vi "get_RL.vi"(8 "error in":errorcluster, 9 "Simulation mode":bool, 10 "Average":i32, 11 "Integration Time (ms)":i32) -> (0 "error out":errorcluster, 2 "RL Spectrum":dbl[](array[numeric]), 3 "WL Values":dbl[](array[numeric]))   [LabVIEW 2021]
doc: "Random Laser Project v2.0\nAndré Romero - 2024\nandretec@ifsc.usp.br"
uses:
  Global_v20.vi
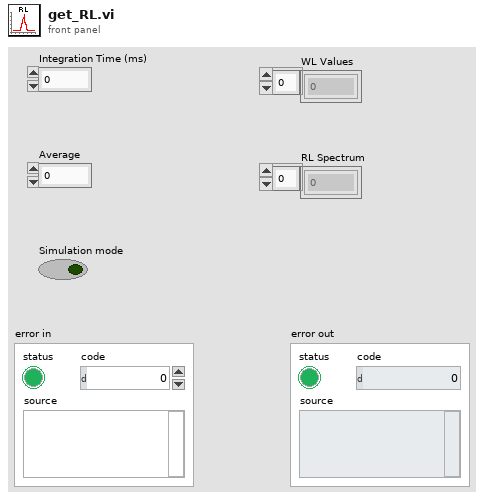
[diagram p1: front panel]
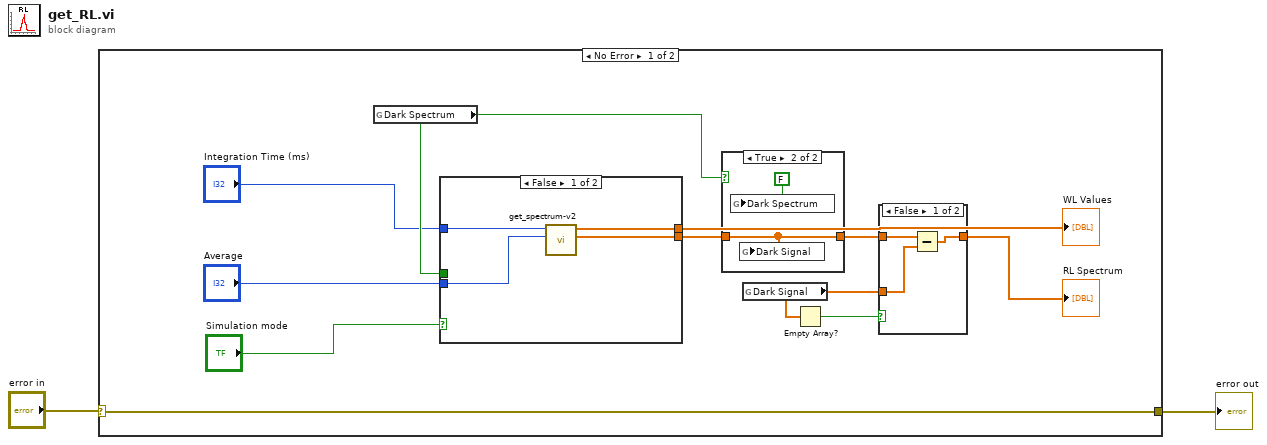
[diagram p0: block diagram]
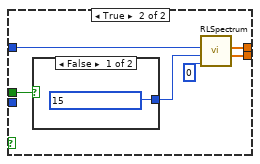
[diagram p3: hidden frame]
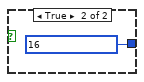
[diagram p4: hidden frame]
diagram:
  n1 = case shown="No Error" "error in" {
    selector: "error in" -> [w3 w33]
    tunnel: [w3 w33] -> w1
    frame No Error {
      n2 = global read "Global_v20.vi" "Dark Spectrum"() -> (w7:bool)
      n3 = case shown="False" "Simulation mode" {
        tunnel: "Integration Time (ms)" -> [w19 w27]
        tunnel: [w21 w26] -> w5
        tunnel: [w20 w25] -> w6
        tunnel: w7 -> [_ w24]
        tunnel: "Average" -> [w18 _]
        frame False {
          n4 = call "get_spectrum-v2.vi"("Average"=w18, "Integration Time (us)"=w19) -> ("Spectrum"=w20:dbl[], "Wavelength (nm)"=w21:dbl[])  [unwired: 7 in, 1 out]
        }
        frame True {
          n5 = case shown="False" w24 {
            tunnel: [u16 15 ("Select Light Source") u16 16 ("Select Light Source")] -> w22
            frame False {
            }
            frame True {
            }
          }
          n6 = call "RLSpectrum.vi"("index (row)"=0, "Select Light Source"=w22, "Integration Time (ms)"=w27) -> ("Spectrum Values"=w25:dbl[], "WL Values"=w26:dbl[])  [unwired: 7 in]
        }
      }
      "WL Values" <- w5
      n7 = case shown="True" w7 {
        tunnel: w6 -> [w30 w32]
        tunnel: [w30 w32] -> w11
        frame False {
        }
        frame True {
          n8 = global write "Global_v20.vi" "Dark Spectrum"(FALSE) -> ()
          n9 = global write "Global_v20.vi" "Dark Signal"(w32) -> ()
        }
      }
      n10 = global read "Global_v20.vi" "Dark Signal"() -> (w13:dbl[])
      n11 = Empty Array?(array=w13) -> (empty?=w10:bool)
      n12 = case shown="False" w10 {
        tunnel: w11 -> [w16 w17]
        tunnel: [w14 w17] -> w12
        tunnel: w13 -> [w15 _]
        frame False {
          n13 = Subtract(x=w16, y=w15) -> (x-y=w14:dbl[])
        }
        frame True {
        }
      }
      "RL Spectrum" <- w12
    }
    frame Error {
    }
  }
  "error out" <- w1
